vi "Rectangle2miniscans.vi"(9 "Apparent Frame Size":dbl=200.0, 10 "Frame Size":dbl=200.0, 11 "X-Y-Z coordinates":T1 {"Apparent Frame Size" format="%#_6f"; "Original FOV (um)" format="%#_6f"; "Pixels per miniscan" format="%#_6f"; "Dwell Time per pixel" format="%#_6f"; "Resolution" format="%#_6f"; "ROI group ID" format="%#_6f"; "Laser Power (%)" format="%#_6f"; "Zoom" format="%#_6f"; "Frame Size" format="%#_6f"; "Number of lines" format="%#_6f"; "Composite ID" format="%#_6f"; "Angle (deg)" format="%#_6f"; "ROI Time (ns)" format="%#_6f"; "ROI ID" format="%#_6f"; "Pixels in ROI" format="%#_6f"; "ROI index" format="%#_6f"; "Z stop" format="%#_6f"; "Y stop" format="%#_6f"; "X stop" format="%#_6f"; "Z start" format="%#_6f"; "X start" format="%#_6f"; "Y start" format="%#_6f"}) -> (0 "No of Miniscans":i32, 1 "No of Pixels in a single miniscan":i32, 2 "XYZ Stop":cluster{"X":dbl, "Y":dbl, "Z":dbl}[](array[cluster]), 3 "XYZ Start":cluster{"X":dbl, "Y":dbl, "Z":dbl}[](array[cluster]), 4 "Zoom":dbl[](array[numeric]))   [LabVIEW 2020]
uses:
  User Interface/Visualisation/Functional Imaging Viewer/Typedefs/ROI parameters data type.ctl
panel:
  out "miniScan Array":dbl[][](array[numeric])
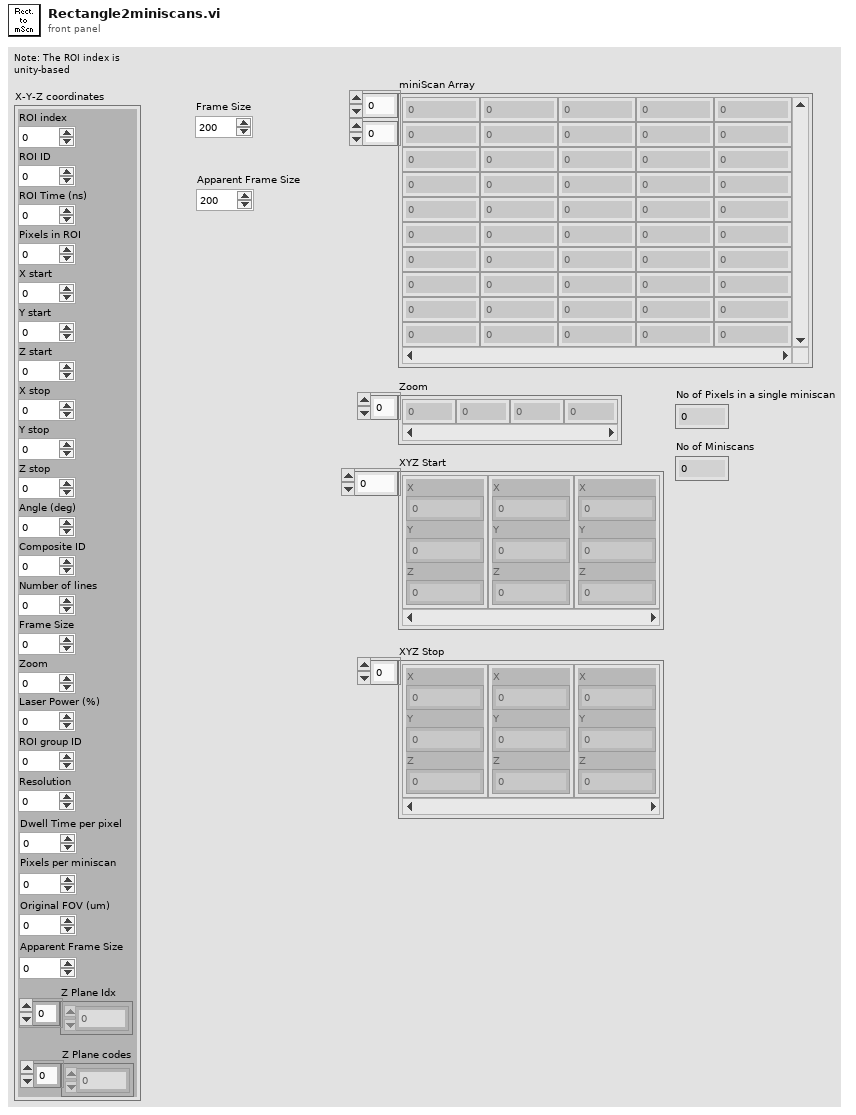
[diagram p1: front panel]
types:
  T1 = typedef "ROI parameters data type.ctl" = cluster{"ROI index":dbl, "ROI ID":dbl, "ROI Time (ns)":dbl, "Pixels in ROI":dbl, "X start":dbl, "Y start":dbl, "Z start":dbl, "X stop":dbl, "Y stop":dbl, "Z stop":dbl, "Angle (deg)":dbl, "Composite ID":dbl, "Number of lines":dbl, "Frame Size":dbl, "Zoom":dbl, "Laser Power (%)":dbl, "ROI group ID":dbl, "Resolution":dbl, "Dwell Time per pixel":dbl, "Pixels per miniscan":dbl, "Original FOV (um)":dbl, "Apparent Frame Size":dbl, "Z Plane Idx":i32[], "Z Plane codes":i32[]}
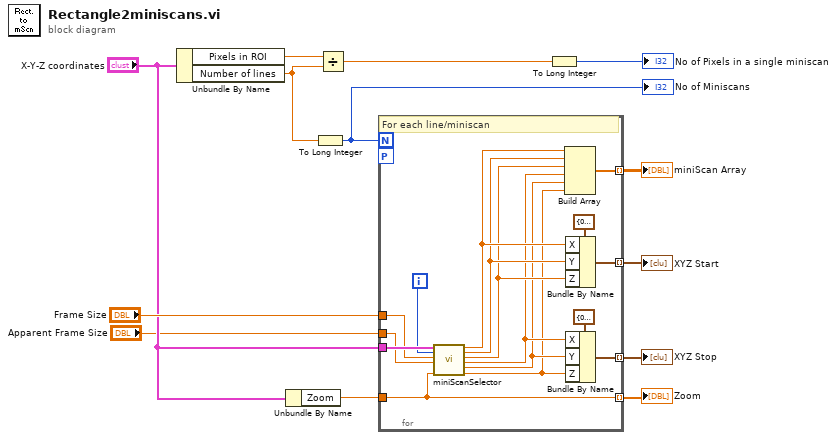
[diagram p0: block diagram]
diagram:
  n1 = Unbundle By Name("X-Y-Z coordinates") -> ("Pixels in ROI"=w6:dbl, "Number of lines"=w9:dbl)
  n2 = Unbundle By Name("X-Y-Z coordinates") -> ("Zoom"=w3:dbl)
  n3 = To Long Integer(number=w9) -> (32bit integer=w7:i32)
  "No of Miniscans" <- w7
  n4 = Divide(x=w6, y=w9) -> (x/y=w4:dbl)
  n5 = for {
    N: w7 -> [_]
    tunnel: [w29] -> w13 mode=indexing
    tunnel: [w28] -> w12 mode=indexing
    tunnel: [w26] -> w11 mode=indexing
    tunnel: "Frame Size" -> [w15]
    tunnel: w3 -> [w17]
    tunnel: [w17] -> w5 mode=indexing
    tunnel: "X-Y-Z coordinates" -> [w24]
    workers-P: _ -> [_]
    tunnel: "Apparent Frame Size" -> [w14]
    i -> [w16]
    # "For each line/miniscan"
    n6 = call "miniScanSelector.vi"("X-Y-Z coordinates"=w24, "index"=w16, "FrameSize"=w15, "App. FrameSize"=w14, "Main zoom"=w17) -> ("Norm X Start"=w23:dbl, "Norm Y Start"=w22:dbl, "Norm Z Start"=w21:dbl, "Norm X Stop"=w20:dbl, "Norm Y Stop"=w19:dbl, "Norm Z Stop"=w18:dbl)  [unwired: 9 in]
    n7 = Build Array(w23, w22, w21, w20, w19, w18) -> (w29:dbl[])
    n8 = Bundle By Name(cluster=cluster{"X":dbl, "Y":dbl, "Z":dbl} {"X"=0.0, "Y"=0.0, "Z"=0.0} ("XYZ"), "X"=w23, "Y"=w22, "Z"=w21) -> (w28:cluster{"X":dbl, "Y":dbl, "Z":dbl})
    n9 = Bundle By Name(cluster=cluster{"X":dbl, "Y":dbl, "Z":dbl} {"X"=0.0, "Y"=0.0, "Z"=0.0} ("XYZ"), "X"=w20, "Y"=w19, "Z"=w18) -> (w26:cluster{"X":dbl, "Y":dbl, "Z":dbl})
  }
  "miniScan Array" <- w13
  "XYZ Stop" <- w11
  "XYZ Start" <- w12
  "Zoom" <- w5
  n10 = To Long Integer(number=w4) -> (32bit integer=→"No of Pixels in a single miniscan":i32)
